vi "Configure EOST List.vi"(8 "error in (no error)":errorcluster {"code" format="%.0x"}, 9 "End Of Step List":i32[](array[numeric]), 10 "Channel Name (1)":string="1", 11 "VISA resource name":refnum<visa-resource-name>) -> (0 "error out":errorcluster {"code" format="%.0x"}, 3 "VISA resource name out":refnum<visa-resource-name>)   [LabVIEW 2018, in "Agilent N6700 Series.lvlib"]
doc: "Configures which list steps generate a trigger out signal at the end of the list step's dwell time.\n\n<b>Note:</b>\nThis VI only applies to models N676xA, N678xA SMU, or models N673xA. N674xA, N675xA, and N677xA with Option 054 (High Speed Test Extensions)."
uses:
  Agilent N6700 Series.lvlib
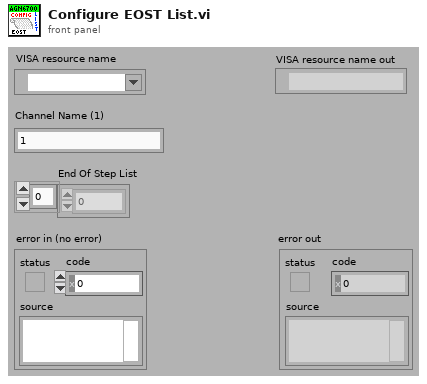
[diagram p1: front panel]
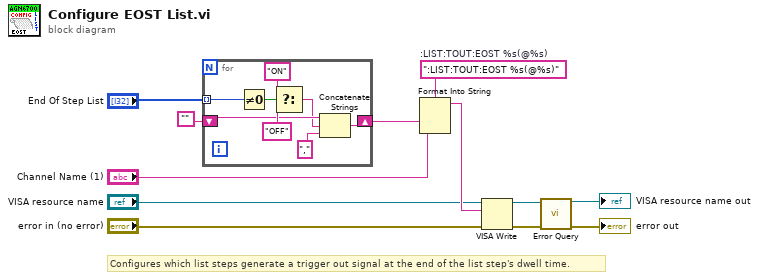
[diagram p0: block diagram]
diagram:
  w12 = ":LIST:TOUT:EOST %s(@%s)"  # :LIST:TOUT:EOST %s(@%s)
  # "Configures which list steps generate a trigger out signal at the end of the list step's dwell time."
  n1 = for {
    tunnel: "End Of Step List" -> [w20] mode=indexing
    shift-right: [w16] -> w5
    shift-left: "" -> [w15]
    n2 = Not Equal To 0?(x=w20) -> (x != 0?=w19:bool)
    n3 = Select(t="ON", s=w19, f="OFF") -> (s? t:f=w14:string)
    n4 = Concatenate Strings(w15, w14, ",") -> (w16:string)
  }
  n5 = Format Into String(format string=w12, w5, "Channel Name (1)") -> (resulting string=w11:string)  [unwired: 2 in, 1 out]
  n6 = VISA Write(VISA resource name="VISA resource name", write buffer=w11, error in (no error)="error in (no error)") -> (VISA resource name out=w2:refnum<visa-resource-name>, error out=w1:errorcluster)  [unwired: 1 out]
  n7 = call "Error Query.vi"("VISA resource name"=w2, "error in (no error)"=w1) -> ("VISA resource name out"=→"VISA resource name out":refnum<visa-resource-name>, "error out"=→"error out":errorcluster)  [unwired: 10 in, 2 out]
